vi "Check Connection.vi"(4 "local port (0)":u16, 6 "timeout [ms]":i32=100, 8 "error in (no error)":errorcluster, 9 "remote port":u16, 10 "ip address":string, 11 "GenNet Variant Protocol in":refnum<class "GenNet Variant Protocol.lvclass">) -> (0 "error out":errorcluster, 3 "GenNet Variant Protocol out":refnum<class "GenNet Variant Protocol.lvclass">)   [LabVIEW 2020, in "hse-gennet.lvlib" / "GenNet Variant Protocol.lvclass"]
doc: "____\nHAMPEL SOFTWARE ENGINEERING v3.8.0 (2023-12-18 14:41)"
uses:
  GenNet Variant Protocol.lvclass
  GenNet Protocol.lvclass
  GenNet Variant Protocol.lvclass/GenNet Variant Protocol.ctl
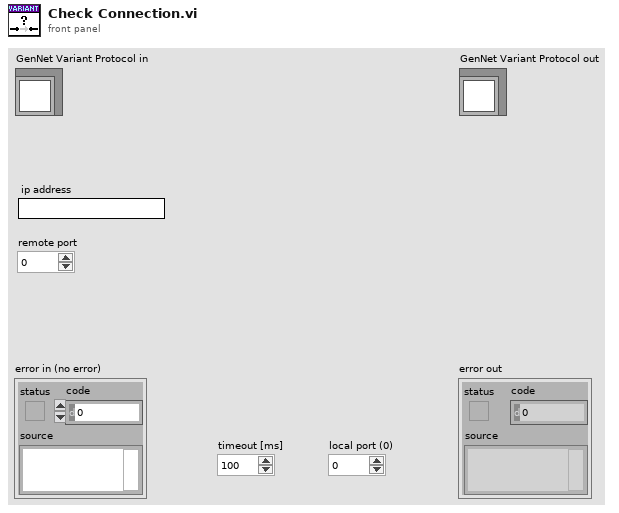
[diagram p1: front panel]
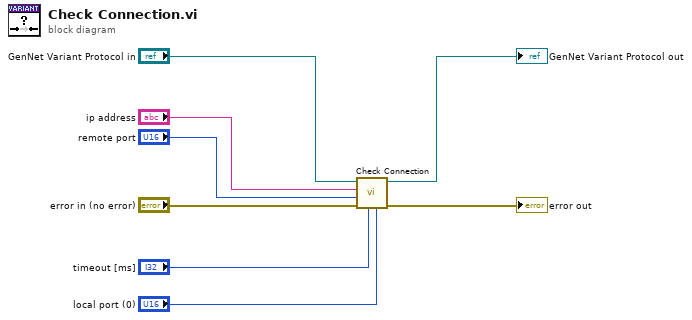
[diagram p0: block diagram]
diagram:
  n1 = call-parent "Check Connection.vi"("local port (0)"="local port (0)", "timeout [ms]"="timeout [ms]", "error in (no error)"="error in (no error)", "remote port"="remote port", "ip address"="ip address", "GenNet Protocol in"="GenNet Variant Protocol in") -> ("error out"=→"error out":errorcluster, "GenNet Protocol out"=→"GenNet Variant Protocol out":refnum<class "GenNet Variant Protocol.lvclass">)  [unwired: 4 in]
